vi "Dispense.vi"(8 "error in (no error)":errorcluster, 10 "BallsIn":i32, 11 "object in":refnum<class "SoldState.lvclass">) -> (0 "error out":errorcluster, 2 "BallsOut":i32, 3 "object out":refnum<class "State.lvclass">)   [LabVIEW 2020, in "SoldState.lvclass"]
uses:
  SoldState.lvclass
  C:/Projects/OpenGDS_DesignPatterns/State1/State_class/State.lvclass
  State_class/State.lvclass
  SoldOutState_class/SoldOutState.lvclass
  NoMoneyState_class/NoMoneyState.lvclass
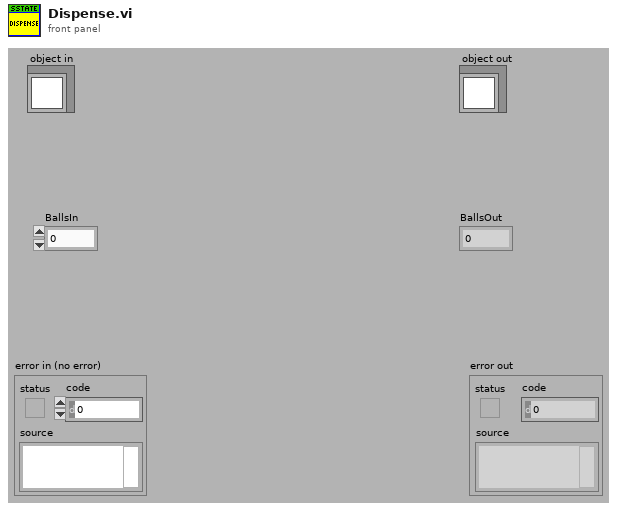
[diagram p1: front panel]
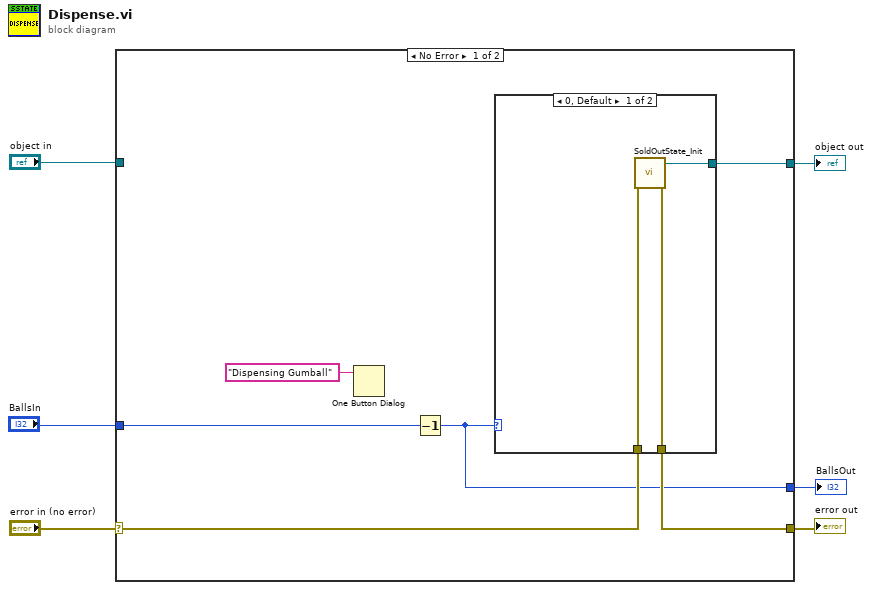
[diagram p0: block diagram]
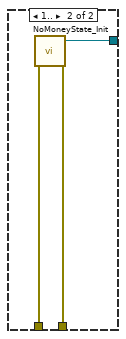
[diagram p2: hidden frame]
diagram:
  n1 = case shown="No Error" "error in (no error)" {
    selector: "error in (no error)" -> [w10 w21]
    tunnel: [w9 w21] -> w5
    tunnel: [w11 w20] -> w3
    tunnel: "object in" -> [_ w20]
    tunnel: "BallsIn" -> [w12 w19]
    tunnel: [w8 w19] -> w1
    frame No Error {
      n2 = One Button Dialog(message="Dispensing Gumball" ("TextIn")) -> ()  [unwired: 1 in, 1 out]
      n3 = Decrement(x=w12) -> (x-1=w8:i32)
      n4 = case shown="0, Default" w8 {
        tunnel: [w15 w18] -> w11
        tunnel: w10 -> [w14 w17]
        tunnel: [w13 w16] -> w9
        frame 0, Default {
          n5 = call "SoldOutState_Init.vi"("error in (no error)"=w14) -> ("error out"=w13:errorcluster, "object out"=w15:refnum<class "SoldOutState.lvclass">)  [unwired: 9 in]
        }
        frame 1.. {
          n6 = call "NoMoneyState_Init.vi"("error in (no error)"=w17) -> ("error out"=w16:errorcluster, "object out"=w18:refnum<class "NoMoneyState.lvclass">)  [unwired: 9 in]
        }
      }
    }
    frame Error {
    }
  }
  "error out" <- w5
  "object out" <- w3
  "BallsOut" <- w1
